vi "tb_interpolation_fft_simio_host.vi"() -> ()   [LabVIEW 2010]
uses:
  <vilib>/rvi/interface/nirviOpenFPGA/nirviOpenFPGA.xnode
  <vilib>/userDefined/High Color/nirio_resource_hc.ctl
  Host Code/Session/Session Handle.ctl
  tb_interpolation_fft_simio_fpga.vi
  <vilib>/rvi/interface/nirviMethod/nirviMethod.xnode
  <vilib>/rvi/interface/nirviCloseFPGA/nirviCloseFPGA.xnode
  <vilib>/rvi/interface/nirviReadWriteControl/nirviReadWriteControl.xnode
  FFT Block/FFT/Controls/FFT States.ctl
  <vilib>/rvi/FXPMathLib/FxpInterpret/XNode/nifxpmath_Interpret.xnode
  <vilib>/Analysis/NI_AALBase.lvlib
  <vilib>/Analysis/1siggen.llb/Ramp Pattern by Samples.vi
  <vilib>/gmath/NI_Gmath.lvlib
  <vilib>/Analysis/NI_AALPro.lvlib
  <vilib>/Analysis/2dsp.llb/Real FFT.vi
  <vilib>/RVI Host/nirviSupport.llb/nirviErrorClusterFromErrorCode.vi
  <vilib>/rvi/errors/niLvFpgaWhatHappensToTopLevelVI.ctl
  <vilib>/rvi/interface/common/niFpgaNodeNameForErrorReporting.ctl
  <vilib>/rvi/errors/niLvFpgaAdjustHostInterfaceError.vi
  <vilib>/FPGAPlugInAG/PXIe-7965R/niLvFpga_Close_PXIe-7965R.vi
  FFT Block/FFT/Controls/FFT Parameters.ctl
panel:
  out "System Waveform Graph":dbl[](graph)
  out "FFT from FPGA 2":dbl[](graph)
  out "Re_FFT2":dbl[](array[numeric])
  out "Re_FFT1":dbl[](array[numeric])
  out "Re FFT2":dbl[](graph)
  out "FFT^2":dbl[](graph)
  out "FFT from FPGA":dbl[](graph)
  out "Input Data":i16(graph)
  in  "Signal Type":T1(ring)
  out "FFT of Resampled Waveform":dbl[](graph)
  out "Resampled Points":dbl[](array[numeric])
  in  "Initial Waveform Size":dbl=1600.0
  in  "Resample Waveform Size":i32=1024
  out "Resampled Wfm Size":i32=1024
  out "Resampled Waveform":dbl[](graph)=[0.0, 0.006141871178498451, 0.01228352190755505, 0.01842469131510103, 0.024565176145137996, 0.030704744928201713, 0.03684311858867577, 0.04298018812771578, 0.04911550567122417, 0.055249113100737025, 0.061380494658199246, 0.06750966126976926, 0.07363624392248455, 0.07976002618999338, 0.08588091321937362, 0.09199836844142179, 0.09811262702226561, 0.10422285040492815, 0.11032940143834599, 0.11643163653659054, 0.12252953998209506, 0.12862289364172555, 0.13471121078360393, 0.14079479114857268, 0.1468725847389934, 0.1529452645137016, 0.15901183578348502, 0.16507262067532258, 0.17112714116401967, 0.17717509817528893, 0.18321668171138306, 0.18925087980900496, 0.1952784950671197, 0.201298152369248, 0.2073106473872674, 0.21331510691686656, 0.219311556136885, 0.2252999390508429, 0.23127941937268354, 0.23725084917768013, 0.24321244009962156, 0.2491655629232505, 0.2551088265391817, 0.26104271524154177, 0.2669667923968709, 0.2728805335141981, 0.2787845571289038, 0.2846772402829921, 0.29056001801530124, 0.29643106424501897, 0.30229145500703614, 0.30814024051714006, 0.31397734216724266, 0.3198030108994681, 0.32561592486299656, 0.33141751425312477, 0.33720545554410447, 0.3429815464038248, 0.34874419400399886, 0.35449389717866575, 0.36023040763953906, 0.3659528380162897, 0.37166237170968086, 0.3773566483523692, 0.3830377927159525, 0.3887036158764725, 0.3943553226501644, 0.3999920367876987, 0.4056134359538412, 0.4112202160490454, 0.4168104422317523, 0.4223861684945501, 0.4279446602375571, 0.4334879532987338, 0.4390144181248012, 0.44452442466745745, 0.45001805369651265, 0.45549392550200435, 0.4609539146533615, 0.46639480873061095, 0.4718194705802251, 0.47722543755435926, 0.4826138953670118, 0.487984185691539, 0.49333560997115056, 0.4986694376204446, 0.5039830045427167, 0.5092790363244974, 0.514554480358579, 0.5198114573581402, 0.5250484500610753, 0.5302655630356752, 0.5354633378949971, 0.5406397837074178, 0.5457974236352466, 0.5509325616838321, 0.5560483681148823, 0.5611423514680791, 0.5662155369063462, 0.5712676199867497, 0.5762974034642231, 0.5813068468187472, 0.5862924540144675, 0.5912576603069355, 0.5961991877803946, 0.6011190947209113, 0.6060161172067335, 0.6108899674377122, 0.615741768181713, 0.6205688113994345, 0.6253742655468141, 0.6301541733261437, 0.6349117333106471, 0.6396446139328351, 0.64435354740495, 0.6490387081443123, 0.653698290202183, 0.6583350453079461, 0.6629445586078884, 0.6675310023939298, 0.672090964270154, 0.6766263014262193, 0.6811361337868848, 0.6856196661507348, 0.6900787089108493, 0.6945097462543743, 0.6989166199765837, 0.7032952068869166, 0.7076485881208082, 0.7119747288602993, 0.7162739474716548, 0.7205470088455688, 0.7247914029956145, 0.7290105837457992, 0.7331996758137725, 0.7373630768766964, 0.7414975033927309, 0.7456044838988861, 0.7496836397330982, 0.7537335674544147, 0.7577568555555124, 0.7617491070017436, 0.7657148537905152, 0.7696498989979583, 0.7735570713560281, 0.7774347570784463, 0.7812827535551802, 0.7851025122340198, 0.7888907404419505, 0.7926515231420261, 0.7963798896905909, 0.800080052118648, 0.8037490767661621, 0.8073880493589352, 0.8109971950924205, 0.8145744176584252, 0.8181231562170326, 0.8216380780219659, 0.8251244102715415, 0.8285779698247947, 0.8320012111419366, 0.8353930509708828, 0.8387526743938778, 0.8420822980485178, 0.8453777863590753, 0.8486438622845801, 0.8518755522852123, 0.8550767525440551, 0.8582449964844509, 0.8613808283171619, 0.8644851624791006, 0.8675551431378807, 0.8705949425397722, 0.8735987699667422, 0.8765720286222044, 0.8795108013292202, 0.8824170615903815, 0.8852903494512121, 0.888129163931638, 0.8909365463915867, 0.8937074780344818, 0.8964473146535081, 0.8991511663166202, 0.9018224981430829, 0.904459411350003, 0.9070618271844492, 0.9096314159828628, 0.9121645151807791, 0.9146658795426059, 0.9171297959916324, 0.9195612755107475, 0.9219569240473301, 0.9243181444701067, 0.926645174460266, 0.9289357722938248, 0.9311938431331356, 0.9334134657007631, 0.9356006111048549, 0.9377505523589931, 0.9398662251464139, 0.9419463809861709, 0.9439902554864759, 0.9460003214467778, 0.9479720829858579, 0.9499108627920582, 0.9518111097942686, 0.9536773352855207, 0.9555067594395581, 0.9573001433688518, 0.9590584769137843, 0.9607787431903182, 0.9624655836705497, 0.9641126124873568, 0.9657259507713823, 0.9673012506645389, 0.9688408384588857, 0.9703441788683063, 0.9718097791749799, 0.9732409400584687, 0.9746323272110831, 0.9759898044662422, 0.9773080587746414, 0.9785910126358319, 0.9798365720523958, 0.9810448050517943, 0.982217487270375, 0.9833508133841524, 0.9844499273589737, 0.9855086914272922, 0.9865326465527521, 0.987518115151642, 0.9884667538545054, 0.9893787827520503, 0.9902519589943333, 0.9910904146928535, 0.991887993994087, 0.9926510629351498, 0.993374613207368, 0.9940619090767191, 0.9947115933561993, 0.9953230103712011, 0.9958987335643675, 0.9964341775637152, 0.9969349537042286, 0.997395243845509, 0.9978199300190885, 0.9982060648788575, 0.9985545957534289, 0.9988665188186147, 0.9991388407257984, 0.9993764008746544, 0.9995725772737115, 0.9997338708987834, 0.9998557402667286, 0.9999407426070804, 0.99998828711618, 0.9999969850953943, 0.999970197781532, 0.9999025900097039, 0.9998001936859306, 0.9996575715473528, 0.9994788886629041, 0.9992619664549267, 0.9990070245494819, 0.9987158340227732, 0.9983846723155791, 0.998018774643303, 0.9976119254600608, 0.9971698866522364, 0.996688899996775, 0.9961707881583606, 0.9956157344372352, 0.9950216293242499, 0.9943925897699529, 0.9937225827773164, 0.9930180027327555, 0.9922738435840296, 0.991493516806549, 0.990675629220793, 0.989819675855998, 0.9889281795414822, 0.9879967313176994, 0.9870309086070006, 0.9860249569498526, 0.9849838535094193, 0.9839046487913852, 0.9827884249346951, 0.9816361251177602, 0.980444952663444, 0.979219667348204, 0.9779537886391212, 0.9766538274434661, 0.9753153069154702, 0.973940870024911, 0.9725299036006794, 0.971081202607071, 0.9695979967982543, 0.9680752546675363, 0.9665188317197044, 0.9649234775828276, 0.9632933610227307, 0.9616263445610037, 0.9599227853632456, 0.9581843505710215, 0.9564076109584138, 0.9545975949412701, 0.9527483656724429, 0.9508655740446376, 0.9489455989377705, 0.946990321593508, 0.9449998816730396, 0.942972419608087, 0.9409118061978743, 0.9388124714636744, 0.9366804750702851, 0.9345111018005761, 0.9323077103029562, 0.9300689564308466, 0.9277945090422534, 0.9254867022418816, 0.9231415490582761, 0.9207642775063248, 0.9183495290435497, 0.9159020846792799, 0.9134191685087112, 0.9109019281368821, 0.9083512076750938, 0.9057645587901028, 0.9031463937497028, 0.9004907480910394, 0.8978037619557464, 0.8950812879177357, 0.8923258943884542, 0.8895369904559591, 0.8867136137104292, 0.8838586880779551, 0.8809677627060851, 0.8780461873907638, 0.8750892041558146, 0.8721007362292967, 0.8690788207071783, 0.8660239202477611, 0.8629375147431371, 0.8598166520036629, 0.8566658724675364, 0.8534798635835138, 0.8502638295945957, 0.8470145064636705, 0.8437337131517806, 0.8404215513682872, 0.837076503781383, 0.833701988124403, 0.8302932011515841, 0.826855528858285, 0.8233848238072029, 0.8198841848416277, 0.816352409017633, 0.8127893422908256, 0.8091970126219904, 0.8055720666062518, 0.8019190922654261, 0.7982334415167749, 0.79451940928906, 0.7907745689179613, 0.7870000505829727, 0.7831965687075733, 0.7793621453086432, 0.7755005786183845, 0.7716068403739834, 0.7676862605771265, 0.7637353002621061, 0.7597562875712127, 0.7557487068574767, 0.7517118738146376, 0.747648259269471, 0.7435542272724663, 0.7394343262848363, 0.7352845728609427, 0.7311083999651639, 0.7269041522646142, 0.7226723503711381, 0.718414223750961, 0.7141274442901292, 0.7098158158578505, 0.7054749648052915, 0.7011093292380278, 0.6967162111040026, 0.692297240494129, 0.687852498283905, 0.6833808728921562, 0.6788851571565782, 0.6743615653083432, 0.6698145137993706, 0.665240672029263, 0.6606426778029827, 0.6560195625496408, 0.6513713334418114, 0.6466996213679026, 0.6420018729081192, 0.6372817865540836, 0.6325357030821035, 0.6277671602942458, 0.6229742453218569, 0.6181579802047055, 0.6133189352511689, 0.6084556892180654, 0.603571222545206, 0.5986617442052768, 0.5937314422465492, 0.5887776157581339, 0.5838021920405193, 0.5788047879697245, 0.5737850084220874, 0.5687447582128698, 0.5636813955576027, 0.5585984219563753, 0.5534928705518123, 0.5483674589841587, 0.5432209632213659, 0.538053902718213, 0.5328672158664292, 0.5276593018374286, 0.5224330255120997, 0.5171852171527059, 0.5119192649258987, 0.5066332213739319, 0.5013284039225404, 0.4960048988751853, 0.4906620328282533, 0.4853018454582088, 0.4799217532724313, 0.47452496660727994, 0.46910917794851825, 0.4636763814522334, 0.4582259303732429, 0.45275796038723015, 0.4472736446442402, 0.441771342896985, 0.4362536691563514, 0.43071817867484774, 0.4251674169130111, 0.41960012737651387, 0.41401713210384333, 0.40841885837225206, 0.4028044890356711, 0.3971760504976804, 0.391531171349649, 0.3858726755228548, 0.38019887176990064, 0.3745111418621821, 0.36880929185080746, 0.3630932034414854, 0.35736414172298264, 0.35162057473481384, 0.34586477460949616, 0.34009497840300257, 0.3343129975459911, 0.3285181450364883, 0.32271087354368366, 0.3168918128969453, 0.31106014473757077, 0.305217649424669, 0.2993625605380959, 0.2934969861309151, 0.2876198773699738, 0.28173212683839605, 0.27583385840996905, 0.2699248381199274, 0.26400627332366666, 0.25807689289897323, 0.2521385364132236, 0.24619007018495567, 0.24023269298784536, 0.23426615480766066, 0.22829067398920672, 0.2223069371507784, 0.21631427257369976, 0.21031407962863377, 0.20430528704410061, 0.19828926388298249, 0.19226552058109303, 0.1862345933256022, 0.18019678097406597, 0.17415187802829296, 0.16810088035122783, 0.16204293226013672, 0.15597935192807458, 0.14990957421663959, 0.14383431680629352, 0.13775362574828778, 0.13166762649181762, 0.1255769120885576, 0.11948110786345043, 0.11338114680911877, 0.10727659076766767, 0.10116820118882584, 0.09505590774543443, 0.08894002997641526, 0.08282089375862088, 0.07669846928049422, 0.07057337101070012, 0.06444535721310139, 0.05831509451910919, 0.05218253361528743, 0.04604805019828529, 0.03991183978243937, 0.03377407998965091, 0.027635118189390444, 0.02149502687010649, 0.015354190431559687, 0.009212734576888596, 0.003070952667687864, -0.003070952667687862, -0.00921273457688895, -0.015354190431560253, -0.0214950268701067, -0.027635118189390295, -0.033774079989651054, -0.03991183978243987, -0.04604805019828571, -0.05218253361528749, -0.05831509451910913, -0.06444535721310168, -0.07057337101070074, -0.07669846928049448, -0.08282089375862078, -0.08894002997641534, -0.09505590774543488, -0.10116820118882631, -0.1072765907676678, -0.11338114680911865, -0.11948110786345066, -0.1255769120885582, -0.13166762649181796, -0.13775362574828776, -0.14383431680629352, -0.14990957421663995, -0.1559793519280751, -0.16204293226013688, -0.16810088035122767, -0.17415187802829313, -0.1801967809740665, -0.18623459332560258, -0.19226552058109306, -0.19828926388298243, -0.20430528704410092, -0.21031407962863438, -0.21631427257369998, -0.2223069371507783, -0.22829067398920683, -0.2342661548076611, -0.2402326929878458, -0.24619007018495576, -0.2521385364132235, -0.2580768928989735, -0.2640062733236673, -0.2699248381199277, -0.275833858409969, -0.2817321268383961, -0.28761987736997424, -0.2934969861309157, -0.299362560538096, -0.30521764942466884, -0.31106014473757093, -0.3168918128969459, -0.32271087354368405, -0.32851814503648824, -0.33431299754599103, -0.3400949784030029, -0.3458647746094968, -0.35162057473481406, -0.3573641417229825, -0.3630932034414855, -0.36880929185080796, -0.37451114186218254, -0.3801988717699007, -0.3858726755228547, -0.39153117134964927, -0.39717605049768107, -0.4028044890356714, -0.40841885837225195, -0.41401713210384333, -0.4196001273765143, -0.4251674169130116, -0.43071817867484785, -0.4362536691563512, -0.4417713428969852, -0.4472736446442408, -0.4527579603872305, -0.45822593037324283, -0.4636763814522334, -0.46910917794851864, -0.4745249666072805, -0.4799217532724315, -0.4853018454582086, -0.4906620328282535, -0.4960048988751858, -0.5013284039225409, -0.5066332213739319, -0.5119192649258986, -0.5171852171527062, -0.5224330255121002, -0.5276593018374288, -0.532867215866429, -0.5380539027182131, -0.5432209632213664, -0.5483674589841592, -0.5534928705518124, -0.5585984219563753, -0.5636813955576029, -0.5687447582128704, -0.5737850084220877, -0.5788047879697245, -0.5838021920405194, -0.5887776157581344, -0.5937314422465498, -0.5986617442052771, -0.6035712225452059, -0.6084556892180656, -0.6133189352511694, -0.6181579802047059, -0.622974245321857, -0.6277671602942458, -0.6325357030821038, -0.6372817865540842, -0.6420018729081194, -0.6466996213679025, -0.6513713334418115, -0.6560195625496412, -0.6606426778029831, -0.6652406720292632, -0.6698145137993706, -0.6743615653083436, -0.6788851571565788, -0.6833808728921565, -0.687852498283905, -0.6922972404941291, -0.6967162111040031, -0.7011093292380284, -0.7054749648052917, -0.7098158158578504, -0.7141274442901294, -0.7184142237509615, -0.7226723503711385, -0.7269041522646142, -0.7311083999651639, -0.7352845728609432, -0.7394343262848369, -0.7435542272724666, -0.7476482592694709, -0.7517118738146378, -0.7557487068574772, -0.7597562875712133, -0.7637353002621062, -0.7676862605771265, -0.7716068403739837, -0.7755005786183852, -0.7793621453086433, -0.7831965687075736, -0.7870000505829728, -0.7907745689179617, -0.7945194092890602, -0.7982334415167753, -0.801919092265426, -0.8055720666062521, -0.8091970126219907, -0.8127893422908262, -0.816352409017633, -0.8198841848416277, -0.823384823807203, -0.8268555288582857, -0.8302932011515843, -0.8337019881244029, -0.837076503781383, -0.840421551368288, -0.843733713151781, -0.8470145064636706, -0.8502638295945955, -0.8534798635835144, -0.856665872467537, -0.8598166520036631, -0.8629375147431368, -0.8660239202477614, -0.8690788207071787, -0.8721007362292971, -0.8750892041558145, -0.878046187390764, -0.8809677627060853, -0.8838586880779555, -0.8867136137104292, -0.8895369904559592, -0.8923258943884543, -0.895081287917736, -0.8978037619557465, -0.9004907480910397, -0.9031463937497027, -0.9057645587901028, -0.9083512076750944, -0.9109019281368825, -0.9134191685087113, -0.9159020846792799, -0.9183495290435502, -0.9207642775063253, -0.9231415490582763, -0.9254867022418815, -0.9277945090422537, -0.930068956430847, -0.9323077103029566, -0.9345111018005761, -0.9366804750702853, -0.9388124714636747, -0.9409118061978747, -0.9429724196080871, -0.9449998816730398, -0.9469903215935083, -0.9489455989377709, -0.9508655740446379, -0.9527483656724431, -0.9545975949412701, -0.9564076109584139, -0.9581843505710217, -0.9599227853632458, -0.9616263445610038, -0.9632933610227307, -0.9649234775828276, -0.9665188317197047, -0.9680752546675364, -0.9695979967982543, -0.9710812026070709, -0.9725299036006796, -0.9739408700249111, -0.9753153069154702, -0.976653827443466, -0.9779537886391213, -0.9792196673482041, -0.980444952663444, -0.9816361251177601, -0.9827884249346952, -0.9839046487913853, -0.9849838535094193, -0.9860249569498527, -0.9870309086070006, -0.9879967313176994, -0.9889281795414823, -0.9898196758559982, -0.990675629220793, -0.9914935168065491, -0.9922738435840297, -0.9930180027327556, -0.9937225827773164, -0.994392589769953, -0.99502162932425, -0.9956157344372353, -0.9961707881583608, -0.9966888999967751, -0.9971698866522364, -0.9976119254600609, -0.9980187746433031, -0.9983846723155793, -0.9987158340227733, -0.999007024549482, -0.9992619664549268, -0.9994788886629042, -0.999657571547353, -0.9998001936859309, -0.999902590009704, -0.9999701977815321, -0.9999969850953944, -0.9999882871161802, -0.9999407426070805, -0.9998557402667286, -0.9997338708987835, -0.9995725772737116, -0.9993764008746546, -0.9991388407257985, -0.9988665188186147, -0.998554595753429, -0.9982060648788577, -0.9978199300190888, -0.997395243845509, -0.9969349537042286, -0.9964341775637153, -0.9958987335643678, -0.9953230103712012, -0.9947115933561993, -0.9940619090767191, -0.9933746132073682, -0.9926510629351502, -0.9918879939940871, -0.9910904146928535, -0.9902519589943334, -0.9893787827520505, -0.9884667538545057, -0.9875181151516421, -0.9865326465527522, -0.9855086914272924, -0.984449927358974, -0.9833508133841525, -0.9822174872703751, -0.9810448050517943, -0.979836572052396, -0.9785910126358321, -0.9773080587746417, -0.9759898044662421, -0.9746323272110832, -0.9732409400584692, -0.9718097791749801, -0.9703441788683062, -0.9688408384588857, -0.9673012506645391, -0.9657259507713827, -0.9641126124873568, -0.9624655836705496, -0.9607787431903184, -0.9590584769137847, -0.9573001433688519, -0.955506759439558, -0.9536773352855205, -0.9518111097942689, -0.9499108627920584, -0.9479720829858579, -0.9460003214467776, -0.9439902554864756, -0.9419463809861711, -0.939866225146414, -0.9377505523589931, -0.9356006111048546, -0.9334134657007631, -0.9311938431331359, -0.9289357722938251, -0.9266451744602656, -0.9243181444701065, -0.9219569240473303, -0.9195612755107478, -0.9171297959916321, -0.9146658795426055, -0.9121645151807791, -0.9096314159828632, -0.907061827184449, -0.9044594113500027, -0.9018224981430828, -0.8991511663166205, -0.8964473146535084, -0.8937074780344818, -0.8909365463915865, -0.8881291639316382, -0.8852903494512122, -0.8824170615903816, -0.8795108013292202, -0.8765720286222044, -0.8735987699667421, -0.8705949425397725, -0.8675551431378808, -0.8644851624791006, -0.8613808283171617, -0.8582449964844511, -0.8550767525440555, -0.8518755522852123, -0.8486438622845796, -0.8453777863590752, -0.8420822980485181, -0.8387526743938776, -0.8353930509708825, -0.8320012111419364, -0.8285779698247949, -0.8251244102715415, -0.8216380780219656, -0.8181231562170321, -0.8145744176584253, -0.8109971950924205, -0.8073880493589352, -0.803749076766162, -0.8000800521186479, -0.7963798896905908, -0.7926515231420265, -0.7888907404419505, -0.7851025122340196, -0.7812827535551798, -0.7774347570784464, -0.7735570713560285, -0.7696498989979583, -0.7657148537905146, -0.7617491070017435, -0.7577568555555128, -0.7537335674544149, -0.7496836397330976, -0.7456044838988858, -0.7414975033927311, -0.7373630768766969, -0.7331996758137722, -0.7290105837457987, -0.7247914029956146, -0.7205470088455693, -0.7162739474716547, -0.711974728860299, -0.7076485881208081, -0.7032952068869169, -0.6989166199765838, -0.6945097462543743, -0.6900787089108491, -0.6856196661507349, -0.6811361337868849, -0.6766263014262194, -0.6720909642701539, -0.6675310023939292, -0.6629445586078881, -0.6583350453079464, -0.6536982902021832, -0.6490387081443116, -0.6443535474049495, -0.6396446139328352, -0.6349117333106475, -0.6301541733261433, -0.6253742655468136, -0.6205688113994346, -0.6157417681817136, -0.610889967437712, -0.6060161172067332, -0.6011190947209111, -0.5961991877803949, -0.5912576603069355, -0.5862924540144674, -0.5813068468187469, -0.5762974034642232, -0.5712676199867496, -0.5662155369063463, -0.561142351468079, -0.5560483681148822, -0.5509325616838318, -0.5457974236352467, -0.5406397837074178, -0.5354633378949971, -0.5302655630356747, -0.5250484500610754, -0.5198114573581405, -0.5145544803585792, -0.5092790363244968, -0.5039830045427166, -0.49866943762044497, -0.4933356099711509, -0.4879841856915385, -0.48261389536701155, -0.4772254375543595, -0.4718194705802249, -0.4663948087306106, -0.46095391465336105, -0.4554939255020044, -0.45001805369651243, -0.44452442466745734, -0.43901441812480096, -0.4334879532987337, -0.42794466023755673, -0.4223861684945501, -0.41681044223175223, -0.4112202160490453, -0.40561343595384064, -0.3999920367876986, -0.39435532265016454, -0.38870361587647256, -0.3830377927159518, -0.377356648352369, -0.37166237170968114, -0.3659528380162899, -0.3602304076395384, -0.35449389717866536, -0.34874419400399903, -0.3429815464038252, -0.33720545554410397, -0.3314175142531242, -0.32561592486299656, -0.31980301089946866, -0.3139773421672424, -0.3081402405171397, -0.3022914550070359, -0.2964310642450193, -0.2905600180153011, -0.28467724028299185, -0.2787845571289036, -0.27288053351419833, -0.26696679239687077, -0.26104271524154177, -0.25510882653918165, -0.24916556292325054, -0.24321244009962123, -0.23725084917768036, -0.23127941937268368, -0.22529993905084206, -0.2193115561368845, -0.21331510691686661, -0.20731064738726773, -0.2012981523692474, -0.19527849506711906, -0.18925087980900485, -0.1832166817113835, -0.17717509817528848, -0.17112714116401917, -0.1650726206753223, -0.1590118357834853, -0.1529452645137014, -0.1468725847389931, -0.14079479114857227, -0.13471121078360404, -0.12862289364172533, -0.12252953998209495, -0.11643163653659035, -0.11032940143834594, -0.10422285040492775, -0.09811262702226572, -0.0919983684414218, -0.08588091321937355, -0.07976002618999281, -0.07363624392248452, -0.06750966126976947, -0.06138049465819937, -0.05524911310073629, -0.049115505671223976, -0.042980188127716125, -0.0368431185886761, -0.03070474492820107, -0.024565176145137636, -0.018424691315101202, -0.01228352190755558, -0.006141871178498006, -6.055890155488852e-08]
  in  "FFT Parameters":T2={"Direction"=TRUE, "scale_sch"=683.0, "Flush Length"=1500} {"scale_sch" format="%.0b"}
  in  "stop":bool
  out "timed out?":bool
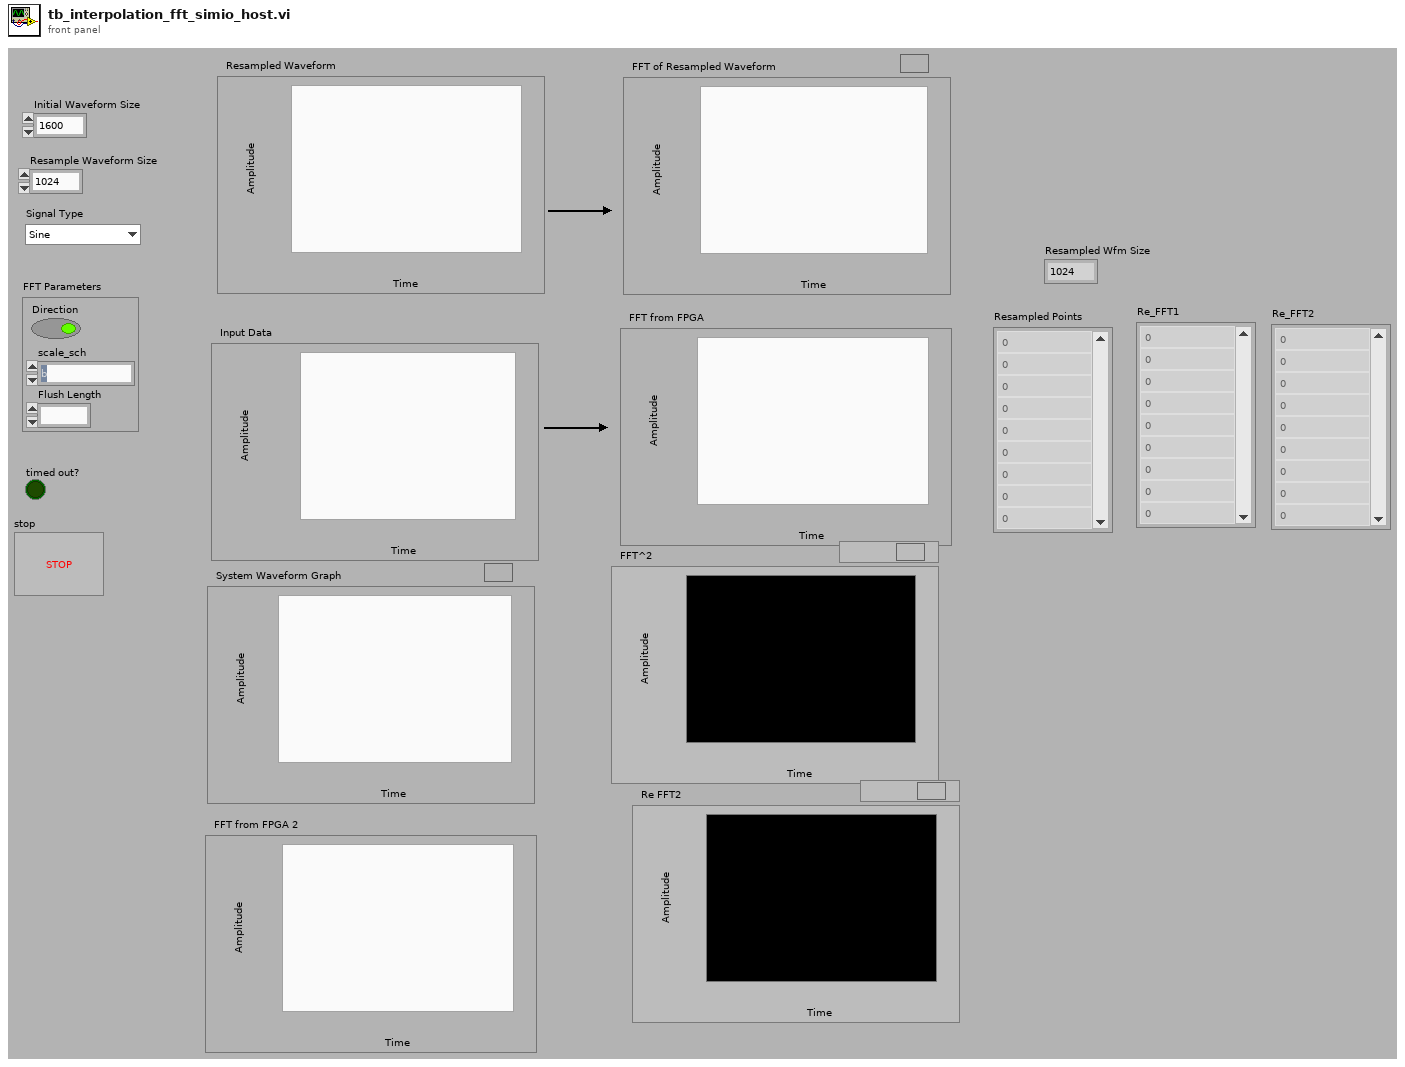
[diagram p1: front panel]
types:
  T1 = enum16{"Sine", "Square", "Chirp", "Rect Pulse", "Triangle Pulse"}
  T2 = typedef "FFT Parameters.ctl" = cluster{"Direction":bool, "scale_sch":fxp<+,10,10>, "Flush Length":u16}
  T3 = typedef "nirio_resource_hc.ctl" = tag
  T4 = typedef "Session Handle.ctl" = refnum<k20>
  T5 = typedef "FFT States.ctl" = enum8{"Configure", "Start FFT processing", "Process", "Unload Last FFT", "Reset"}
  T6 = typedef "niFpgaNodeNameForErrorReporting.ctl" = enum16{"Open FPGA VI Reference", "Read/Write Control", "Invoke Method: Abort", "Invoke Method: Acknowledge IRQ", "Invoke Method: Download", "Invoke Method: FIFO.Configure", "Invoke Method: FIFO.Read", "Invoke Method: FIFO.Start", "Invoke Method: FIFO.Stop", "Invoke Method: FIFO.Write", "Invoke Method: Reset", "Invoke Method: Run", "Invoke Method: Wait on IRQ", "Close FPGA VI Reference"}
  T7 = typedef "niLvFpgaWhatHappensToTopLevelVI.ctl" = enum16{"top level VI scripted behind XNode", "top level VI inlined behind XNode"}
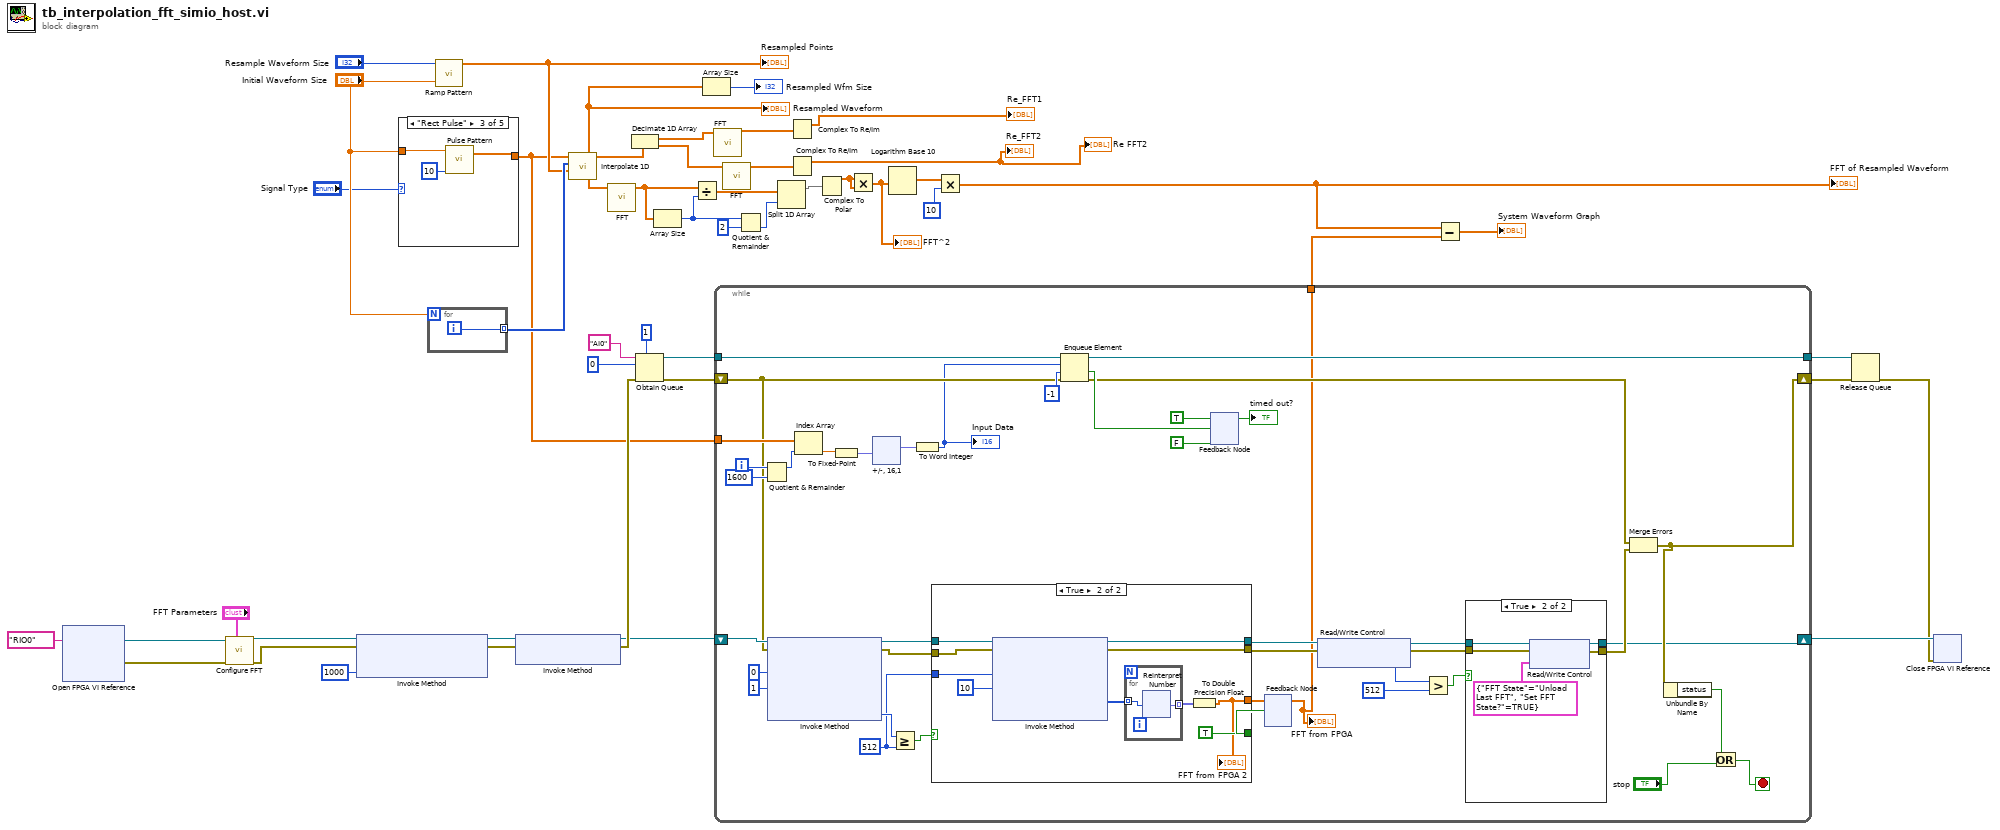
[diagram p0: block diagram]
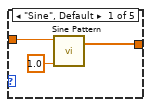
[diagram p2: hidden frame]
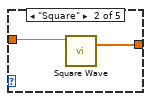
[diagram p3: hidden frame]
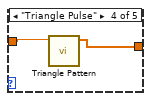
[diagram p4: hidden frame]
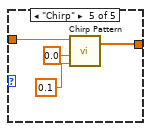
[diagram p5: hidden frame]
diagram:
  n1 = xnode "Open FPGA VI Reference"("resource name"=T3 "RIO0") -> ("FPGA VI Reference Out"=w40:T4, "error out"=w39:errorcluster)  [unwired: 1 in]
  n2 = call "Configure FFT.vi"("FFT Parameters"="FFT Parameters", "error in"=w39, "FPGA Session"=w40) -> ("error out"=w35:errorcluster, "FPGA Session"=w36:T4)  [unwired: 7 in]
  n3 = xnode "Invoke Method"("FPGA VI Reference In"=w36, "error in"=w35, "Depth"=u32 1000) -> ("FPGA VI Reference Out"=w33:T4, "error out"=w32:errorcluster)
  n4 = case shown="\"Rect Pulse\"" "Signal Type" {
    tunnel: "Initial Waveform Size" -> [w50 w52 w55 w57 w61]
    tunnel: [w49 w51 w54 w56 w60] -> w19
    frame "Sine", Default {
      n5 = call <vilib>:"Sine Pattern.vi"("cycles"=1.0, "samples"=w50) -> ("Sinusoidal Pattern"=w49:dbl[])  [unwired: 2 in, 1 out]
    }
    frame "Square" {
      n6 = call <vilib>:"Square Wave.vi"("samples"=w52) -> ("square wave"=w51:dbl[])  [unwired: 5 in, 2 out]
    }
    frame "Rect Pulse" {
      n7 = call <vilib>:"Pulse Pattern.vi"("width"=10, "samples"=w55) -> ("Pulse Pattern"=w54:dbl[])  [unwired: 2 in, 1 out]
    }
    frame "Triangle Pulse" {
      n8 = call <vilib>:"Triangle Pattern.vi"("samples"=w57) -> ("Triangle Pattern"=w56:dbl[])  [unwired: 9 in, 1 out]
    }
    frame "Chirp" {
      n9 = call <vilib>:"Chirp Pattern.vi"("f2"=0.1, "f1"=0.0, "samples"=w61) -> ("Chirp Pattern"=w60:dbl[])  [unwired: 1 in, 1 out]
    }
  }
  n10 = for {
    N: "Initial Waveform Size" -> [_]
    tunnel: [w62] -> w26 mode=indexing
    i -> [w62]
  }
  n11 = call-poly <vilib>:"Ramp Pattern.vi"("end"="Initial Waveform Size", "samples"="Resample Waveform Size") -> ("Ramp Pattern"=w24:dbl[])  [unwired: 8 in, 1 out]
  "Resampled Points" <- w24
  n12 = xnode "Invoke Method"("FPGA VI Reference In"=w33, "error in"=w32) -> ("FPGA VI Reference Out"=w30:T4, "error out"=w31:errorcluster)
  n13 = call <vilib>:"Interpolate 1D.vi"("xi"=w24, "X"=w26, "Y"=w19) -> ("yi"=w9:dbl[])  [unwired: 6 in, 2 out]
  "Resampled Waveform" <- w9
  n14 = call-poly <vilib>:"FFT.vi"("X"=w9) -> ("FFT {X}"=w15:cdb[])  [unwired: 9 in, 1 out]
  n15 = Decimate 1D Array(w9) -> (w8:dbl[], w7:dbl[])
  n16 = Obtain Queue(max queue size (-1, unlimited)=1, name (unnamed)="AI0", element data type=i16 0, error in (no error)=w31) -> (queue out=w45:refnum<queue>, error out=w43:errorcluster)  [unwired: 1 in, 1 out]
  n17 = Array Size(array=w15) -> (size(s)=w14:i32)
  n18 = Divide(x=w15, y=w14) -> (x/y=w16:cdb[])
  n19 = Array Size(array=w9) -> (size(s)=→"Resampled Wfm Size":i32)
  n20 = call-poly <vilib>:"FFT.vi"("X"=w8) -> ("FFT {X}"=w6:cdb[])  [unwired: 9 in, 1 out]
  n21 = while {
    tunnel: w45 -> [w103]
    shift-right: [w82] -> w41
    shift-left: w43 -> [w91]
    tunnel: w19 -> [w102]
    tunnel: [w98] -> w42
    shift-right: [w71] -> w29
    shift-left: w30 -> [w92]
    tunnel: [w63] -> w11
    i -> [w101]
    stop <- w79 stop-if-true
    w84 = u32 512 ("y")
    n22 = Quotient & Remainder(x=w101, y=1600) -> (x-y*floor(x/y)=w99:i32)  [unwired: 1 out]
    n23 = xnode "Invoke Method"("FPGA VI Reference In"=w92, "error in"=w91, "Number of Elements"=u32 0, "Timeout (ms)"=1) -> ("FPGA VI Reference Out"=w88:T4, "error out"=w87:errorcluster, "Elements Remaining"=w86:u32)  [unwired: 1 out]
    n24 = Index Array(array=w102, index=w99) -> (element=w69:dbl)
    n25 = To Fixed-Point(number=w69) -> (fixed-point=w68:fxp<+/-,16,1>)  [unwired: 1 in]
    n26 = xnode "+/-, 16,1"("x"=w68) -> ("y"=w67:fxp<+/-,16,16>)
    n27 = Greater Or Equal?(x=w86, y=w84) -> (x >= y?=w85:bool)
    n28 = To Word Integer(number=w67) -> (16bit integer=w66:i16)
    "Input Data" <- w66
    n29 = case shown="True" w85 {
      tunnel: w88 -> [w159 w169]
      tunnel: w87 -> [w158 w168]
      tunnel: w84 -> [_ w167]
      tunnel: [w158 w165] -> w77
      tunnel: [w159 w164] -> w78
      tunnel: [_ w160] -> w65
      tunnel: [_ TRUE] -> w64
      frame False {
      }
      frame True {
        n30 = xnode "Invoke Method"("FPGA VI Reference In"=w169, "error in"=w168, "Number of Elements"=w167, "Timeout (ms)"=10) -> ("FPGA VI Reference Out"=w164:T4, "error out"=w165:errorcluster, "Data"=w163:i16[])  [unwired: 1 out]
        n31 = for {
          tunnel: w163 -> [w171] mode=indexing
          tunnel: [w170] -> w162 mode=indexing
          n32 = xnode "Reinterpret Number"("x"=w171) -> ("y"=w170:fxp<+/-,16,8>)
        }
        n33 = To Double Precision Float(number=w162) -> (double precision float=w160:dbl[])
        "FFT from FPGA 2" <- w160
      }
    }
    n34 = Enqueue Element(queue=w103, element=w66, timeout in ms (-1)=-1, error in (no error)=w91) -> (queue out=w98:refnum<queue>, timed out?=w96:bool, error out=w83:errorcluster)
    n35 = feedback-in #1(TRUE, w96) -> ()
    n36 = feedback #1(FALSE) -> (→"timed out?":bool)
    n37 = feedback-in #2(w65, w64) -> ()
    n38 = feedback #2() -> (w63:dbl[])  [unwired: 1 in]
    "FFT from FPGA" <- w63
    n39 = xnode "Read/Write Control"("FPGA VI Reference In"=w78, "error in"=w77) -> ("FPGA VI Reference Out"=w74:T4, "error out"=w73:errorcluster, "FFT Input Valids"=w76:u64)
    n40 = Greater?(x=w76, y=u64 512) -> (0:w70:bool)
    n41 = case shown="True" w70 {
      tunnel: w74 -> [w110 w115]
      tunnel: w73 -> [w109 w114]
      tunnel: [w109 w112] -> w72
      tunnel: [w110 w111] -> w71
      frame False {
      }
      frame True {
        n42 = xnode "Read/Write Control"("FPGA VI Reference In"=w115, "error in"=w114, "FFT State"=cluster{"FFT State":T5, "Set FFT State?":bool} {"FFT State"=enum."Unload Last FFT", "Set FFT State?"=TRUE}) -> ("FPGA VI Reference Out"=w111:T4, "error out"=w112:errorcluster)
      }
    }
    n43 = Merge Errors(w83, w72) -> (w82:errorcluster)
    n44 = Unbundle By Name(w82) -> ("status"=w81:bool)
    n45 = Or(x=w81, y="stop") -> (x .or. y?=w79:bool)
  }
  n46 = call-poly <vilib>:"FFT.vi"("X"=w7) -> ("FFT {X}"=w5:cdb[])  [unwired: 9 in, 1 out]
  n47 = Quotient & Remainder(x=w14, y=2) -> (floor(x/y)=w22:i32)  [unwired: 1 out]
  n48 = Split 1D Array(array=w16, index=w22) -> (first subarray=w10:cdb[])  [unwired: 1 out]
  n49 = Complex To Re/Im(x + iy=w6) -> (x=→"Re_FFT1":dbl[])  [unwired: 1 out]
  n50 = Complex To Re/Im(x + iy=w5) -> (x=→"Re FFT2" →"Re_FFT2":dbl[])  [unwired: 1 out]
  n51 = Complex To Polar(r * e^(i*theta)=w10) -> (r=w12:dbl[])  [unwired: 1 out]
  n52 = Multiply(x=w12, y=w12) -> (x*y=w1:dbl[])
  "FFT^2" <- w1
  n53 = Logarithm Base 10(1:w1) -> (0:w18:dbl[])
  n54 = Multiply(x=w18, y=10) -> (x*y=w13:dbl[])
  "FFT of Resampled Waveform" <- w13
  n55 = Subtract(x=w13, y=w11) -> (x-y=→"System Waveform Graph":dbl[])
  n56 = Release Queue(queue=w42, error in (no error)=w41) -> (error out=w28:errorcluster)  [unwired: 1 in, 2 out]
  n57 = xnode "Close FPGA VI Reference"("FPGA VI Reference In"=w29, "error in"=w28) -> ()  [unwired: 1 out]
